vi "读内部参数解析.vi"(9 "读取的字节":i32, 10 "响应":string="$RPARA:FF,FF,3B9ACA00,00e9,03F3,0000,0001,FFFF,0C;\\r\\n") -> (2 "读内部参数":string[](array[string]))   [LabVIEW 2020]
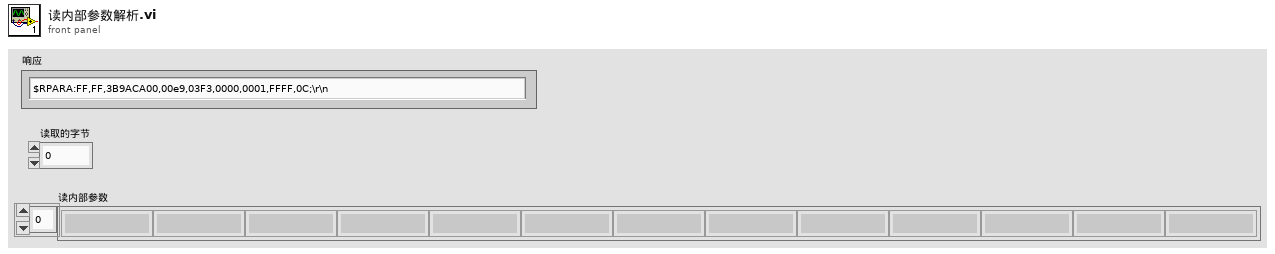
[diagram p1: front panel]
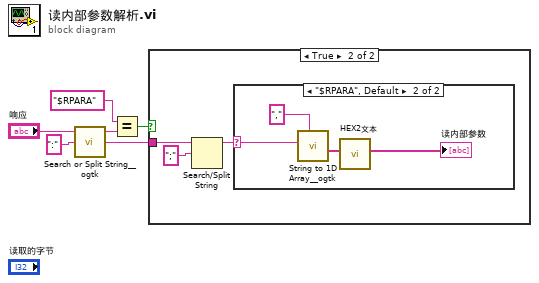
[diagram p0: block diagram]
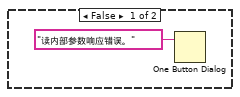
[diagram p2: hidden frame]
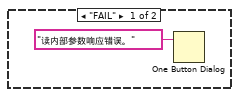
[diagram p3: hidden frame]
diagram:
  n1 = call <userlib>:"Search or Split String__ogtk.vi"("search string/char (-)"=":", "string"="响应") -> ("substring after match"=w1:string, "substring before match"=w4:string)  [unwired: 1 in, 1 out]
  n2 = Equal?(x="$RPARA" ("消息"), y=w4) -> (x = y?=w2:bool)
  n3 = case shown="True" w2 {
    tunnel: w1 -> [_ w9]
    frame False {
      n4 = One Button Dialog(message="读内部参数响应错误。" ("消息")) -> ()  [unwired: 1 in, 1 out]
    }
    frame True {
      n5 = Search/Split String(string=w9, search string/char (-)=";" ("搜索字符串/字符(-)")) -> (substring before match=w8:string)  [unwired: 1 in, 2 out]
      n6 = case shown="\"$RPARA\", Default" w8 {
        selector: w8 -> [_ w12]
        frame "FAIL" {
          n7 = One Button Dialog(message="读内部参数响应错误。" ("消息")) -> ()  [unwired: 1 in, 1 out]
        }
        frame "$RPARA", Default {
          n8 = call <userlib>:"String to 1D Array__ogtk.vi"("delimiter (Tab)"=",", "string"=w12) -> ("Array of Strings"=w14:string[])  [unwired: 9 in]
          n9 = call "HEX2文本.vi"("读内部参数"=w14) -> ("内部参数(文本)"=→"读内部参数":string[])  [unwired: 10 in]
        }
      }
    }
  }
